vi "GapWeight.vi"(11 "GIC Input":T2={"     Use ?\nOff       On"=[FALSE, TRUE, FALSE, TRUE], "Mode:"=FALSE, "Extra Port"="", "Hokuyo Port"="COM7", "Tx Prop  Port"="COM6", "Compass Port"="", "GPS Port"="", "Num of WPs"=0, "WP Lats and Longs"={"WP Lats"=[], "WP Longs"=[]}, "Obst Lats and Longs"={"Obst Lats"=[], "Obst Longs"=[]}, "Parameters"=[], "GPS Data"=[], "Compass"=0.0, "LMS Vector"=[], "Vision Vector"=[], "Direction Cmd"=0.0, "Speed Cmd"=0.0, "WP Vector"=[], "WP Number"=0, "Extra"=0, "SW Map"=[], "Path Cluster"={"Path x node"=[], "Path y node"=[]}, "Sim Course"=[]} {"Obst Lats and Longs"."Obst Longs" format="%#_8g"; "Obst Lats and Longs"."Obst Lats" format="%#_8g"}) -> (3 "GIC Output":T1={"     Use ?\nOff       On"=[FALSE, TRUE, FALSE, TRUE], "Mode:"=FALSE, "Extra Port"="", "Hokuyo Port"="COM7", "Tx Prop Port"="COM6", "Compass Port"="", "GPS Port"="", "Num of WPs"=0, "WP Lats and Longs"={"WP Lats"=[], "WP Longs"=[]}, "Obst Lats and Longs"={"Obst Lats"=[], "Obst Longs"=[]}, "Parameters"=[], "GPS Data"=[], "Compass"=0.0, "LMS Vector"=[], "Vision Vector"=[], "Direction Cmd"=0.0, "Speed Cmd"=0.0, "WP Vector"=[], "WP Number"=0, "Extra"=0, "SW Map"=[], "Path Cluster"={"Path x node"=[], "Path y node"=[]}, "Sim Course"=[]} {"Obst Lats and Longs"."Obst Longs" format="%#_8g"; "Obst Lats and Longs"."Obst Lats" format="%#_8g"})   [LabVIEW 2014]
panel:
  out "nr":dbl
  out "nl":dbl
  out "Wr67":dbl
  out "Wl67":dbl
  out "lr67":dbl
  out "ll67":dbl
  out "sr67":dbl
  out "sl67":dbl
  out "tr67":dbl
  out "tl67":dbl
  out "dr67":dbl
  out "dl67":dbl
  out "Wr90":dbl
  out "Wr45":dbl
  out "Wr23":dbl
  out "W0":dbl
  out "Wl23":dbl
  out "Wl45":dbl
  out "Wl90":dbl
  out "lr90":dbl
  out "lr45":dbl
  out "lr23":dbl
  out "l0":dbl
  out "ll23":dbl
  out "ll45":dbl
  out "ll90":dbl
  out "sr90":dbl
  out "sr45":dbl
  out "sr23":dbl
  out "s0":dbl
  out "sl23":dbl
  out "sl45":dbl
  out "sl90":dbl
  out "tr90":dbl
  out "tr45":dbl
  out "tr23":dbl
  out "t0":dbl
  out "tl23":dbl
  out "tl45":dbl
  out "tl90":dbl
  out "Conf":dbl
  out "Slant":dbl
  out "drW":dbl
  out "dr45W":dbl
  out "dr23W":dbl
  out "d0W":dbl
  out "dl23W":dbl
  out "dl45W":dbl
  out "dlW":dbl
  out "wpvector":dbl[](array[numeric])
  out "ya":dbl
  out "xa":dbl
  out "dl23":dbl
  out "dr23":dbl
  out "a":dbl
  out "s":dbl
  out "objy":dbl
  out "objx":dbl
  out "dl":dbl
  out "dr":dbl
  out "dl45":dbl
  out "dr45":dbl
  out "d0":dbl
  # "GapWeight"
  # "Input:"
  # "Output"
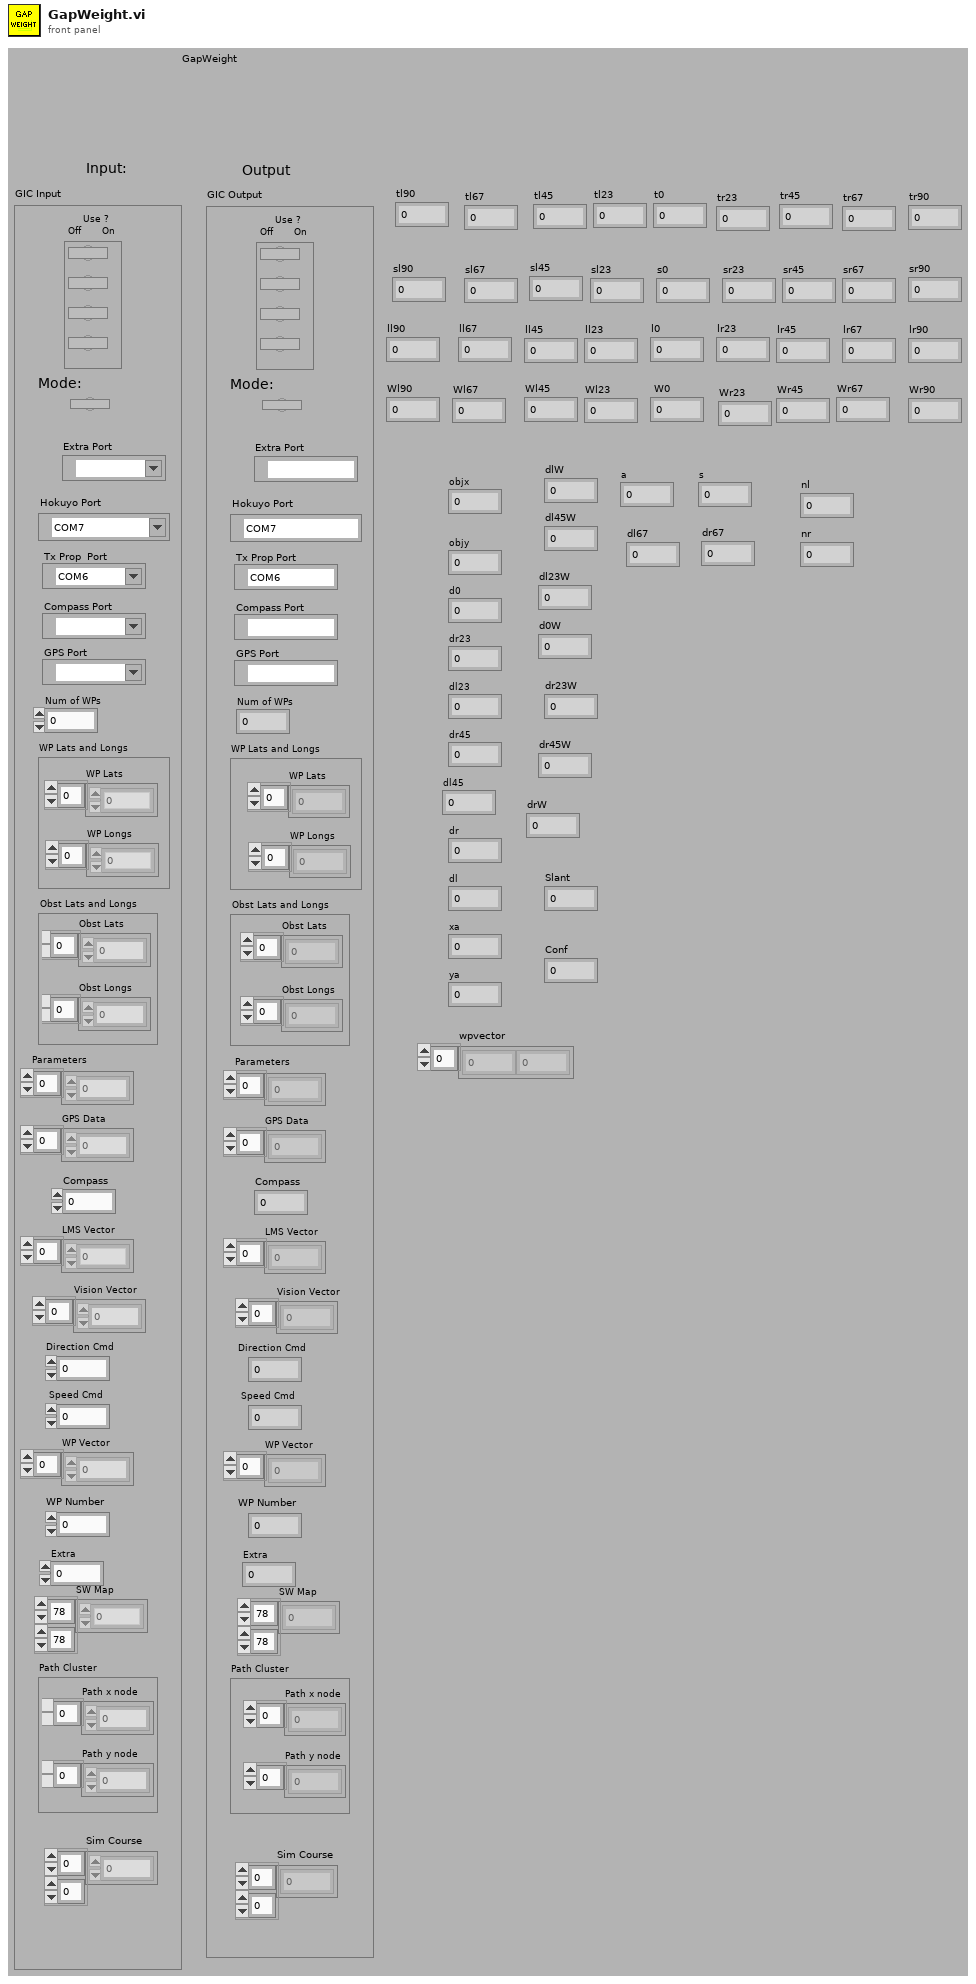
[diagram p1: front panel]
types:
  T1 = cluster{"     Use ?\nOff       On":bool[], "Mode:":bool, "Extra Port":refnum<visa-resource-name>, "Hokuyo Port":refnum<visa-resource-name>, "Tx Prop Port":refnum<visa-resource-name>, "Compass Port":refnum<visa-resource-name>, "GPS Port":refnum<visa-resource-name>, "Num of WPs":i16, "WP Lats and Longs":cluster{"WP Lats":dbl[], "WP Longs":dbl[]}, "Obst Lats and Longs":cluster{"Obst Lats":dbl[], "Obst Longs":dbl[]}, "Parameters":dbl[], "GPS Data":dbl[], "Compass":dbl, "LMS Vector":dbl[], "Vision Vector":dbl[], "Direction Cmd":dbl, "Speed Cmd":dbl, "WP Vector":dbl[], "WP Number":i32, "Extra":i16, "SW Map":i32[][], "Path Cluster":cluster{"Path x node":dbl[], "Path y node":dbl[]}, "Sim Course":i8[][]}
  T2 = cluster{"     Use ?\nOff       On":bool[], "Mode:":bool, "Extra Port":refnum<visa-resource-name>, "Hokuyo Port":refnum<visa-resource-name>, "Tx Prop  Port":refnum<visa-resource-name>, "Compass Port":refnum<visa-resource-name>, "GPS Port":refnum<visa-resource-name>, "Num of WPs":i16, "WP Lats and Longs":cluster{"WP Lats":dbl[], "WP Longs":dbl[]}, "Obst Lats and Longs":cluster{"Obst Lats":dbl[], "Obst Longs":dbl[]}, "Parameters":dbl[], "GPS Data":dbl[], "Compass":dbl, "LMS Vector":dbl[], "Vision Vector":dbl[], "Direction Cmd":dbl, "Speed Cmd":dbl, "WP Vector":dbl[], "WP Number":i32, "Extra":i16, "SW Map":i32[][], "Path Cluster":cluster{"Path x node":dbl[], "Path y node":dbl[]}, "Sim Course":i8[][]}
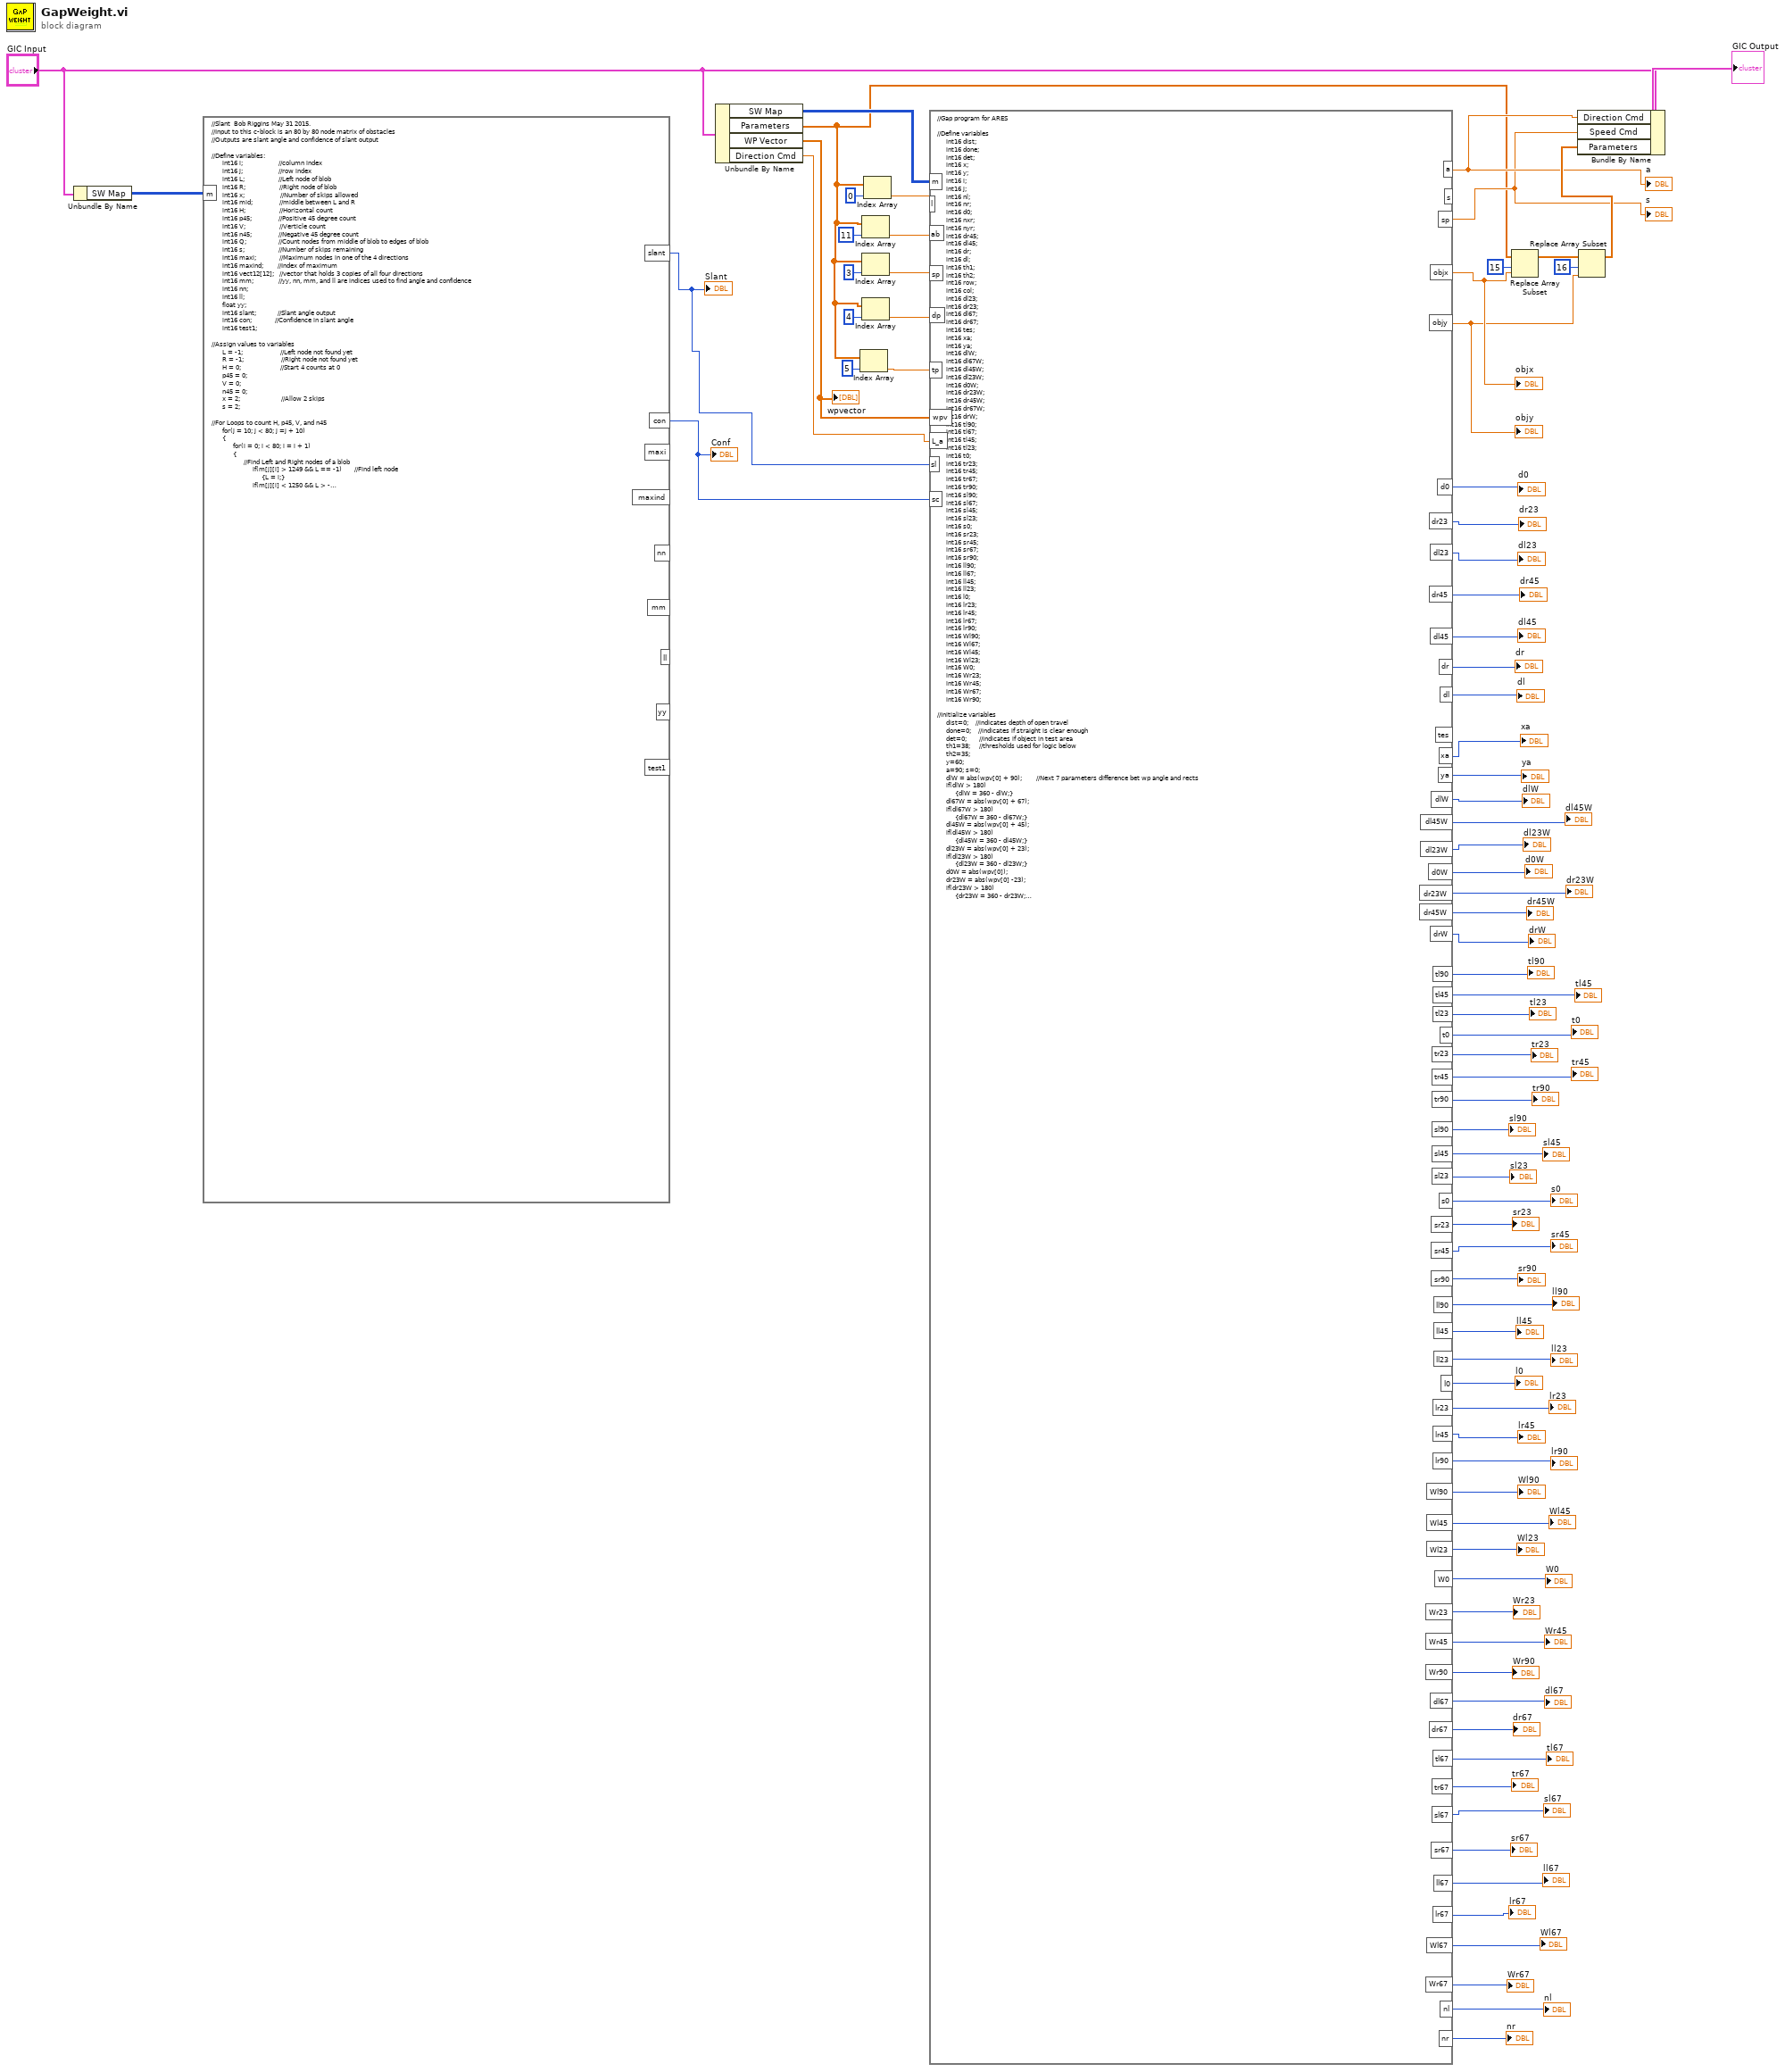
[diagram p0: block diagram]
diagram:
  n1 = Unbundle By Name("GIC Input") -> ("SW Map"=w52:i32[][])
  n2 = formula code="//Slant  Bob Riggins May 31 2015.  \n//Input to this c-block is an 80 by 80 node matrix of obstacles\n//Outputs are slant angle and confidence of slant output\n\n//Define variables:\n      int16 i;                    //column index\n      int16 j;                    //row index\n      int16 L;                   //Left node of blob\n      int16 R;                   //Right node of blob\n      int16 x;                    //Number of skips allowed\n      int16 mid;               //middle between L and R\n      int16 H;                   //Horizontal count\n      int16 p45;               //Positive 45 degree count\n      int16 V;                   //Verticle count\n      int16 n45;               //Negative 45 degree count\n      int16 Q;                  //Count nodes from middle of blob to edges of blob\n      int16 s;                   //Number of skips remaining\n      int16 maxi;             //Maximum nodes in one of the 4 directions\n      int16 maxind;        //Index of maximum\n      int16 vect12[12];   //vector that holds 3 copies of all four directions\n      int16 mm;              //yy, nn, mm, and ll are indices used to find angle and confidence\n      int16 nn;\n      int16 ll;\n      float yy;\n      int16 slant;            //Slant angle output\n      int16 con;             //Confidence in slant angle\n      int16 test1;\n\n//Assign values to variables\n      L = -1;                     //Left node not found yet\n      R = -1;                     //Right node not found yet\n      H = 0;                      //Start 4 counts at 0\n      p45 = 0;\n      V = 0;\n      n45 = 0;\n      x = 2;                       //Allow 2 skips\n      s = 2;\n\n//For Loops to count H, p45, V, and n45\n      for(j = 10; j < 80; j =j + 10)\n      {\n            for(i = 0; i < 80; i = i + 1)\n            {\n                  //Find Left and Right nodes of a blob\n                       if(m[j][i] > 1249 && L == -1)       //Find left node\n                            {L = i;}\n                       if(m[j][i] < 1250 && L > -1 && s == 0)          //Find right node\n                            {R = i - 1 - x;} \n                       if(m[j][i] <1250 && L > -1 && s > 0)         //Allow for skips\n                            {s = s - 1;}\n                       if(i == 79 && m[j][i] > 1249 && L == -1)      //single node at edge\n                       {                                                                            //define L and R there\n                             L == 79;\n                             R == 79;\n                       }       \n                       if(i == 79 && m[j][i] > 1249 && L > -1)       //blob at edge (L found)\n                            {R = 79;}   \n                       if(i == 79 && m[j][i] < 1250 && L > -1)       //blob at edge (L found)\n                            {R = 78;}\n\n                       if(L > -1 && R > -1)         //If L and R exist then start counting from mid\n                       {\n                            H = H + (R - L);                         //Updated H\n                            if(j==10)\n                                 {test1 = R;}\n                            mid = int((L + R)/2);                //Set up middle of blob for counting\n                            L = -1;\n                            R = -1;\n                            s = x;\n                            Q = 1; \n                \n                       //Count N45 (negative 45 degrees thru mid of blob)\n                            while (s > 0 && j + Q < 80 && mid + Q < 80)\n                                {\n                                     while (m[j + Q][mid + Q] > 1249)    //Count down and to right\n                                          {\n                                               n45 = n45 + 1;\n                                               s = x;\n                                               Q = Q + 1;\n                                          }\n                                     while (m[j + Q][mid + Q] < 1250 && s > 0)   //Allow x skips\n                                          {\n                                               n45 = n45 + 1;\n                                               s = s - 1;\n                                               Q = Q + 1;\n                                          }\n                                }     //end of while loop for counting n45 down and to right\n                                n45 = n45 - x;\n                                s = x;\n                                Q = 1;\n\n                                while (s > 0 && j - Q > -1 && mid - Q > -1)\n                                {\n                                     while (m[j - Q][mid - Q] > 1249)    //Count up and to left\n                                          {\n                                               n45 = n45 + 1;\n                                               s = x;\n                                               Q = Q + 1;\n                                          }\n                                     while (m[j - Q][mid - Q] < 1250 && s > 0)   //Allow x skips\n                                          {\n                                               n45 = n45 + 1;\n                                               s = s - 1;\n                                               Q = Q + 1;\n                                          }\n                                }     //end of while loop for counting n45 up and to left\n                                n45 = n45 - x;\n                                s = x;\n                                Q = 1;\n\n                       //Count V (verticle thru mid of blob)\n                            while (s > 0 && j + Q < 80)\n                                {\n                                     while (m[j + Q][mid] > 1249)    //Count down from mid\n                                          {\n                                               V = V + 1;\n                                               s = x;\n                                               Q = Q + 1;\n                                          }\n                                     while (m[j + Q][mid] < 1250 && s > 0)   //Allow x skips\n                                          {\n                                               V = V + 1;\n                                               s = s - 1;\n                                               Q = Q + 1;\n                                          }\n                                }     //end of while loop for counting V down\n                                V = V - x;\n                                s = x;\n                                Q = 1;\n\n                                while (s > 0 && j - Q > -1)\n                                {\n                                     while (m[j - Q][mid] > 1249)    //Count up\n                                          {\n                                               V = V + 1;\n                                               s = x;\n                                               Q = Q + 1;\n                                          }\n                                     while (m[j - Q][mid] < 1250 && s > 0)   //Allow x skips\n                                          {\n                                               V = V + 1;\n                                               s = s - 1;\n                                               Q = Q + 1;\n                                          }\n                                }     //end of while loop for counting V up\n                                V = V - x;\n                                s = x;\n                                Q = 1;\n\n                       //Count p45 (positive 45 degrees thru mid of blob)\n                            while (s > 0 && j + Q < 80 && mid - Q > -1)\n                                {\n                                     while (m[j + Q][mid - Q] > 1249)    //Count down and to left\n                                          {\n                                               p45 = p45 + 1;\n                                               s = x;\n                                               Q = Q + 1;\n                                          }\n                                     while (m[j + Q][mid - Q] < 1250 && s > 0)   //Allow x skips\n                                          {\n                                               p45 = p45 + 1;\n                                               s = s - 1;\n                                               Q = Q + 1;\n                                          }\n                                }     //end of while loop for counting p45 down and to left\n                                p45 = p45 - x;\n                                s = x;\n                                Q = 1;\n\n                                while (s > 0 && j - Q > -1 && mid + Q < 80)\n                                {\n                                     while (m[j - Q][mid + Q] > 1249)    //Count up and to right\n                                          {\n                                               p45 = p45 + 1;\n                                               s = x;\n                                               Q = Q + 1;\n                                          }\n                                     while (m[j - Q][mid + Q] < 1250 && s > 0)   //Allow x skips\n                                          {\n                                               p45 = p45 + 1;\n                                               s = s - 1;\n                                               Q = Q + 1;\n                                          }\n                                }     //end of while loop for counting p45 up and to right\n                                p45 = p45 - x;\n                                s = x;\n                                Q = 1;\n\n                       }                                                    //end of IF for counts for blob\n            }                                    //end of FOR for i\n      }                                          //end of FOR for j\n      \n      //Now have H, p45, V, n45.  Find slan and con  (slant angle and confidence)\n            maxi = H;                                   //Initialize process of finding maximum direction\n            maxind = 0;\n            if(p45 > maxi)\n            {\n                 maxi = p45;\n                 maxind = 1;\n            }\n            if(V > maxi)\n            {\n                 maxi = V;\n                 maxind = 2;\n            }\n            if(n45 > maxi)\n            {\n                 maxi = n45;\n                 maxind = 3;\n            }                                                    //now, max value of 4 directions in maxi\n                                                                 //maxind is index of direction of max\n\n            for(i = 0; i < 3; i = i + 1)            //Next, make vect12, 3 copies of 4 directions\n            {\n                 vect12[4*i] = H;\n                 vect12[4*i + 1] = p45;\n                 vect12[4*i + 2] = V;\n                 vect12[4*i + 3] = n45;\n            }\n           \n            if(maxi != 0)\n            {\n                 nn = vect12[maxind - 1];                          //Use max direction and \"pull\" off to sides\n                 mm = vect12[maxind + 1];\n                 ll = vect12[maxind + 2];\n                 yy = (mm - nn)/(maxi + mm + mm);\n                 con = (1 - (ll/maxi)) * 100;                                    //Confidence of slant calculation\n\n                 if(maxind == 0)                                         //Find slant angle\n                    {slant = 45 * yy;}\n                 if(maxind == 1)                                         \n                    {slant = 45 * (1 - yy);}\n                 if(maxind == 2)                                         \n                    {slant = (45 * (1 - yy)) - 45;}\n                 if(maxind == 3)                                         \n                    {slant = -45 * (1 + yy);}\n             }\n\n             if(maxi == 0)\n             {\n                  slant = 0;\n                  con = 0;\n             }"("m"=w52) -> ("slant"=w51:i16, "con"=w50:i16)  [unwired: 7 out]
  "Slant" <- w51
  "Conf" <- w50
  n3 = Unbundle By Name("GIC Input") -> ("SW Map"=w83:i32[][], "Parameters"=w44:dbl[], "WP Vector"=w49:dbl[], "Direction Cmd"=w1:dbl)
  "wpvector" <- w49
  n4 = Index Array(array=w44, index=5) -> (element=w42:dbl)
  n5 = Index Array(array=w44, index=11) -> (element=w63:dbl)
  n6 = Index Array(array=w44, index=3) -> (element=w47:dbl)
  n7 = Index Array(array=w44, index=4) -> (element=w45:dbl)
  n8 = Index Array(array=w44, index=0) -> (element=w81:dbl)
  n9 = formula code="//Gap program for ARES\n\n//Define variables\n     int16 dist;\n     int16 done;\n     int16 det;\n     int16 x;\n     int16 y;\n     int16 i;\n     int16 j;\n     int16 nl;\n     int16 nr;\n     int16 d0;\n     int16 nxr;\n     int16 nyr;\n     int16 dr45;\n     int16 dl45;\n     int16 dr;\n     int16 dl;\n     int16 th1;\n     int16 th2;\n     int16 row;\n     int16 col;\n     int16 dl23;\n     int16 dr23;\n     int16 dl67;\n     int16 dr67;\n     int16 tes;\n     int16 xa;\n     int16 ya;\n     int16 dlW;\n     int16 dl67W;\n     int16 dl45W;\n     int16 dl23W;\n     int16 d0W;\n     int16 dr23W;\n     int16 dr45W;\n     int16 dr67W;\n     int16 drW;\n     int16 tl90;\n     int16 tl67;\n     int16 tl45;\n     int16 tl23;\n     int16 t0;\n     int16 tr23;\n     int16 tr45;\n     int16 tr67;\n     int16 tr90;\n     int16 sl90;\n     int16 sl67;\n     int16 sl45;\n     int16 sl23;\n     int16 s0;\n     int16 sr23;\n     int16 sr45;\n     int16 sr67;\n     int16 sr90;\n     int16 ll90;\n     int16 ll67;\n     int16 ll45;\n     int16 ll23;\n     int16 l0;\n     int16 lr23;\n     int16 lr45;\n     int16 lr67;\n     int16 lr90;\n     int16 Wl90;\n     int16 Wl67;\n     int16 Wl45;\n     int16 Wl23;\n     int16 W0;\n     int16 Wr23;\n     int16 Wr45;\n     int16 Wr67;\n     int16 Wr90;\n\n//Initialize variables\n     dist=0;    //indicates depth of open travel\n     done=0;    //indicates if straight is clear enough\n     det=0;       //indicates if object in test area\n     th1=38;     //thresholds used for logic below\n     th2=35;\n     y=60;\n     a=90; s=0;\n     dlW = abs(wpv[0] + 90);        //Next 7 parameters difference bet wp angle and rects\n     if(dlW > 180)\n          {dlW = 360 - dlW;}\n     dl67W = abs(wpv[0] + 67);\n     if(dl67W > 180)\n          {dl67W = 360 - dl67W;}\n     dl45W = abs(wpv[0] + 45);\n     if(dl45W > 180)\n          {dl45W = 360 - dl45W;}\n     dl23W = abs(wpv[0] + 23);\n     if(dl23W > 180)\n          {dl23W = 360 - dl23W;}\n     d0W = abs(wpv[0]);\n     dr23W = abs(wpv[0] -23);\n     if(dr23W > 180)\n          {dr23W = 360 - dr23W;}\n     dr45W = abs(wpv[0] -45);\n     if(dr45W > 180)\n          {dr45W = 360 - dr45W;}\n     dr67W = abs(wpv[0] -67);\n     if(dr67W > 180)\n          {dr67W = 360 - dr67W;}\n     drW = abs(wpv[0] - 90);\n     if(drW > 180)\n          {drW = 360 - drW;}\n\n//Count obstacles to immediate left and right for weight info\n//Number of objects on left is nl and on right nr.\n     nl = 0; nr = 0;\n     for(i = 1; i< 10; i = i + 1)\n     {\n          for(j = 1; j< 10; j = j + 1)\n          {\n               if(m[60 - j][40 - i] > 1249)\n               {nl = nl + 1;}\n               if(m[60 - j][40 + i] > 1249)  \n               {nr = nr + 1;}\n          }\n     }   \n\n//Test rectangle in front. Check for obstacles\n     while(det==0 && y>=1)\n     {\n          y=60-dist;\n          x=40-l;\n          while (x<= 40+l && det==0)\n          {\n               if (m[y][x]>=2500)\n                    {det=1;}\n               x=x+1;\n          }\n          dist=dist+1;\n     }\n     d0=dist-1;     //d0 is how far it can move forward\n\n//Test rectangle at 23 degrees to left\n     //Set variables\n          dist=0;det=0;nxr=40;row=0;x=40;y=60;\n     //Check for obstacles\n          while(det==0 && x>2+2*l && y>=1)\n          {\n               x=nxr-l;\n               if(row==0)\n               {\n                    while(x<=nxr+l && det==0)\n                    {\n                         if((y!=60 && y!=59) || x!=40+l)\n                         {\n                              if(m[y][x]>=2500)\n                                   {det=1;}\n                         }\n                         x=x+1;\n                    }\n                    row=1;dist=dist+1;y=y-1;\n               }\n               else\n               {\n                     while(x<=nxr+l && det==0)\n                    {\n                         if((y!=60 && y!=59) || x!=40+l)\n                         {\n                              if(m[y][x]>=2500)\n                                   {det=1;}\n                         } \n                         x=x+1;\n                   }\n                    row=0;dist=dist+1;y=y-1; nxr=nxr-1;\n              }  \n          }  \n          dl23=dist-1;  \n\n//Test rectangle at 23 degrees to right\n     //Set variables\n          dist=0;det=0;nxr=40;row=0;x=40;y=60;\n     //Check for obstacles\n          while(det==0 && x<=77 && y>=1)\n          {\n               x=nxr-l;\n               if(row==0)\n               {\n                    while(x<=nxr+l && det==0)\n                    {\n                         if((y!=60 && y!=59) || x!=40-l)\n                         {\n                              if(m[y][x]>=2500)\n                                   {det=1;}\n                         }\n                         x=x+1;\n                    }\n                    row=1;dist=dist+1;y=y-1;\n               }\n               else\n               {\n                      while(x<=nxr+l && det==0)\n                    {\n                         if((y!=60 && y!=59) || x!=40-l)\n                         {\n                              if(m[y][x]>=2500)\n                                   {det=1;}\n                         }\n                         x=x+1;\n                    }\n                    row=0;dist=dist+1;y=y-1; nxr=nxr+1;\n               }\n          }\n          dr23=dist-1;   \n\n//Test rectangle at 67 degrees to right\n     //Set variables\n          dist=0;det=0;nyr=60;col=0;x=40;y=60;\n     //Check for obstacles\n          while(det==0 && x< 80-l)\n          {\n               y=nyr-l;\n               if(col==0)\n               {\n                    while(y<=nyr+l && det==0)\n                    {\n                         if((x!=40 && x!=39) || y!=60+l)\n                         {\n                              if(m[y][x]>=2500)\n                                   {det=1;}\n                         }\n                         y=y+1;\n                    }\n                    col=1;dist=dist+1;x=x+1;\n               }\n               else\n               {\n                      while(y<=nyr+l && det==0)\n                    {\n                         if((x!=40 && x!=39) || y!=60+l)\n                         {\n                              if(m[y][x]>=2500)\n                                   {det=1;}\n                         }\n                         y=y+1;\n                    }\n                    col=0;dist=dist+1;x=x+1; nyr=nyr-1;\n               }\n          }\n          dr67=(dist-1) * 1.086;   \n\n//If room to the front or 23 degree to either side, just go there\n     //if(d0>=th1 || dr23>=th1 || dl23>=th1)\n          //{done=1;}\n\n//Test rectangle at 45 degrees to right\n     //Set variables\n          dist=0;det=0;nxr=40;nyr=60;x=40;\n     //Check for obstacles\n          while(det==0 && x<=77)\n          {\n               x=nxr-l; y=nyr-l;\n               while(x<=nxr+l && det==0)\n                    {\n                         if(m[y][x]>=2500)\n                              {det=1;}\n                         if(m[y-1][x]>=2500)\n                              {det=1;}\n                         if(x==nxr+l)\n                         {\n                              if(m[y][x+1]>=2500)\n                                   {det=1;}\n                         }\n                         x=x+1; y=y+1;\n                    }\n                    nxr=nxr+1;nyr=nyr-1;\n                    dist=dist+1;\n          }\n          dr45=(dist-1)*1.616;\n\n//Test rectangle at 45 degrees to left\n     //Set variables\n          dist=0;det=0;nxr=40;nyr=60;x=40;\n     //Check for obstacles\n          while(det==0 && x>=2+2*l)\n          {\n               x=nxr-l; y=nyr+l;\n               while(x<=nxr+l && det==0)\n                    {\n                         if(m[y][x]>=2500)\n                              {det=1;}\n                         if(m[y][x-1]>=2500)\n                              {det=1;}\n                         if(x==nxr+l)\n                         {\n                              if(m[y-1][x]>=2500)\n                                   {det=1;}\n                         }\n                         x=x+1; y=y-1;\n                    }\n                    nxr=nxr-1;nyr=nyr-1;\n                    dist=dist+1;\n          }\n          dl45=(dist-1)*1.4886;   \n\n//Test rectangle at 67 degrees to left\n     //Set variables\n          dist=0;det=0;nyr=60;col=0;x=40;y=60;\n     //Check for obstacles\n          while(det==0 && x>l)\n          {\n               y=nyr-l;\n               if(col==0)\n               {\n                    while(y<=nyr+l && det==0)\n                    {\n                         if((x!=40 && x!=39) || y!=60+l)\n                         {\n                              if(m[y][x]>=2500)\n                                   {det=1;}\n                         }\n                         y=y+1;\n                    }\n                    col=1;dist=dist+1;x=x-1;\n               }\n               else\n               {\n                     while(y<=nyr+l && det==0)\n                    {\n                         if((x!=40 && x!=39) || y!=60+l)\n                         {\n                              if(m[y][x]>=2500)\n                                   {det=1;}\n                         } \n                         y=y+1;\n                   }\n                    col=0;dist=dist+1;x=x-1; nyr=nyr-1;\n              }  \n          }  \n          dl67=(dist-1) * 1.086;  \n\n//Test rectangle to the right (right below and above robot)\n     //Set variables\n          dist=0;det=0; x=0;\n          while(det==0 && x<=78)\n          {\n               x=40+dist; y=60+l;\n               while(y>=60-l && det==0)\n               {\n                    if (m[y][x] >=2500)\n                         {det=1;}\n                    y=y-1;\n               }\n               dist=dist+1;\n          }\n          dr=(dist-1)*1.0256;\n\n//Test rectangle to the left (left below and above robot)\n     //Set variables\n          dist=0;det=0; x=1;\n          while(det==0 && x>=1)\n          {\n               x=40-dist; y=60+l;\n               while(y>=60-l && det==0)\n               {\n                    if (m[y][x] >=2500)\n                         {det=1;}\n                    y=y-1;\n               }\n               dist=dist+1;\n          }\n          dl=dist-1;\n\n//If WP dist is less than a rectangle dist that is closest in angle to wp, go that way\n//Else if rect angle that is closest to wp has dist at least th1, go that way\n     if (dlW < dl67W && dlW < dl45W && dlW < dl23W && dlW < d0W && dlW < dr23W && dlW < dr45W && dlW < dr67W && dlW < drW)\n          {\n               if ( dl >= wpv[1] * 10)\n                    {s = dl; a = 90 - wpv[0]; done = 1;}\n          } \n     if (dl67W < dlW && dl67W < dl45W && dl67W < dl23W && dl67W < d0W && dl67W < dr23W && dl67W < dr45W && dl67W < dr67W && dl67W < drW)\n          {\n               if ( dl45 >= wpv[1] * 10)\n                    {s = dl67; a = 90 - wpv[0]; done = 1;}\n          }   \n     if (dl45W < dlW && dl45W < dl67W && dl45W < dl23W && dl45W < d0W && dl45W < dr23W && dl45W < dr45W && dl45W < dr67W && dl45W < drW)\n          {\n               if ( dl45 >= wpv[1] * 10)\n                    {s = dl45; a = 90 - wpv[0]; done = 1;}\n          }   \n     if (dl23W < dlW && dl23W < dl67W && dl23W < dl45W && dl23W < d0W && dl23W < dr23W && dl23W < dr45W && dl23W < dr67W && dl23W < drW)\n          {\n               if ( dl23 >= wpv[1] * 10)\n                    {s = dl23; a = 90 - wpv[0]; done = 1;}\n          } \n     if (d0W < dlW && d0W < dl67W && d0W < dl45W && d0W < dl23W && d0W < dr23W && d0W < dr45W && d0W < dr67W && d0W < drW)\n          {\n               if ( d0 >= wpv[1] * 10)\n                    {s = d0; a = 90 - wpv[0]; done = 1;}\n          } \n     if (dr23W < dlW && dr23W < dl67W && dr23W < dl45W && dr23W < dl23W && dr23W < d0W && dr23W < dr45W && dr23W < dr67W && dr23W < drW)\n          {\n               if ( dr23 >= wpv[1] *  10)\n                    {s = dr23; a = 90 - wpv[0]; done = 1;}\n          } \n     if (dr45W < dlW && dr45W < dl67W && dr45W < dl45W && dr45W < dl23W && dr45W < d0W && dr45W < dr23W && dr45W < dr67W && dr45W < drW)\n          {\n               if ( dr45>= wpv[1] * 10)\n                    {s = dr45; a = 90 - wpv[0]; done = 1;}\n          } \n     if (dr67W < dlW && dr67W < dl67W && dr67W < dl45W && dr67W < dl23W && dr67W < d0W && dr67W < dr23W && dr67W < dr45W && dr67W < drW)\n          {\n               if ( dr45>= wpv[1] * 10)\n                    {s = dr67; a = 90 - wpv[0]; done = 1;}\n          } \n     if (drW < dlW && drW < dl67W && drW < dl45W && drW < dl23W && drW < d0W && drW < dr23W && drW < dr45W && drW < dr67W)\n          {\n               if ( dr>= wpv[1] * 10)\n                    {s = dr; a = 90 - wpv[0]; done = 1;}\n          } \n     if (done ==1)\n          {\n               objx=40+cos(a*0.017453)*s;\n               objy=60-sin(a*0.017453)*s;\n          }\n\n//If no direct path to wp on local map then weight the gaps\n     if(done == 0)\n          {\n               if(nl + nr > 20)\n                    {tp = 0; sp = 0;}\n\n               tl90 = (100 - (dlW*100)/180) * tp;\n               tl67 = (100 - (dl67W*100)/180) * tp;\n               tl45 = (100 - (dl45W*100)/180) * tp;\n               tl23 = (100 - (dl23W*100)/180) * tp;\n               t0 = (100 - (d0W*100)/180) * tp;\n               tr23 = (100 - (dr23W*100)/180) * tp;\n               tr45 = (100 - (dr45W*100)/180) * tp;\n               tr67 = (100 - (dr67W*100)/180) * tp;\n               tr90 = (100 - (drW*100)/180) * tp;\n               \n               if(sc<60)\n                    {sp = 0;;}\n\n               sl90 = ((1 - sin(sl*3.14159/180))*(sc/2)) * sp;\n               sl67= ((-.9205*sin(sl*3.14159/180) + .39073 * cos(sl*3.14159/180) + 1) * (sc/2)) * sp;\n               sl45= ((-.707*sin(sl*3.14159/180) + .707 * cos(sl*3.14159/180) + 1) * (sc/2)) * sp;\n               sl23= ((-.39073*sin(sl*3.14159/180) + .9205 * cos(sl*3.14159/180) + 1) * (sc/2)) * sp;\n               s0 = ((cos(sl*3.14159/180) + 1) * (sc/2)) * sp;\n               sr23= ((.39073*sin(sl*3.14159/180) + .9205 * cos(sl*3.14159/180) + 1) * (sc/2)) * sp;\n               sr45= ((.707*sin(sl*3.14159/180) + .707 * cos(sl*3.14159/180) + 1) * (sc/2)) * sp;\n               sr67= ((.9205*sin(sl*3.14159/180) + .39073 * cos(sl*3.14159/180) + 1) * (sc/2)) * sp;\n               sr90 = ((1 + sin(sl*3.14159/180))*(sc/2)) * sp;\n\n               //ll90 = ((dl * 100)/40) * dp;\n               //ll67 = ((dl67 * 100)/40) * dp;\n               //ll45 = ((dl45 * 100)/57) * dp;\n               //ll23 = ((dl23 * 100)/59) * dp;\n               //l0 = ((d0 * 100)/60) * dp;\n               //lr23 = ((dr23 * 100)/59) * dp;\n               //lr45 = ((dr45 * 100)/57) * dp;\n               //lr67 = ((dr67 * 100)/40) * dp;\n               //lr90 = ((dr * 100)/40) * dp;\n\n               ll90 = (dl * 100)/60 * dp;\n               ll67 = (dl67 * 100)/60 * dp;\n               ll45 = ((dl45 * 100)/60) * dp;\n               ll23 = ((dl23 * 100)/60) * dp;\n               l0 = ((d0 * 100)/60) * dp;\n               lr23 = ((dr23 * 100)/60) * dp;\n               lr45 = ((dr45 * 100)/60) * dp;\n               lr67 = ((dr67 * 100)/60) * dp;\n               lr90 = ((dr * 100)/60) * dp;\n\n               Wl90 = tl90 + sl90 + ll90;\n               Wl67 = tl67 + sl67 + ll67;\n               Wl45 = tl45 + sl45 + ll45;\n               Wl23 = tl23 + sl23 + ll23;\n               W0 = t0 + s0 + l0;\n               Wr23 = tr23 + sr23 + lr23;\n               Wr45 = tr45 + sr45 + lr45;\n               Wr67 = tr67 + sr67 + lr67;\n               Wr90 = tr90 + sr90 + lr90;\n\n          }\n\n           \n//Go in direction of biggest weight at speed proportional to distance\n     if(done == 0)\n          {\n          if(d0>th2 || dr67 > th2 || dr45 >th2 || dl45>th2 || dl67 > th2 || dr>th2 || dl>th2 || dr23>th2 || dl23>th2)\n          {\n               if(Wl90 >= Wl67 && Wl90>=Wl45 && Wl90>=Wl23 && Wl90>= W0 && Wl90>=Wr23 && Wl90>=Wr45 && Wl90>=Wr67 && Wl90>= Wr90)\n                    {s=dl;a=180;}\n               if(Wl67 >= Wl90 && Wl67>=Wl45 && Wl67>=Wl23 && Wl67 >= W0 && Wl67 >=Wr23 && Wl67 >=Wr45 && Wl67 >=Wr67 && Wl67 >= Wr90)\n                    {s=dl67;a=157 + (dl - dl45)/3;}\n               if(Wl45>=Wl90 && Wl45 >= Wl67 && Wl45>=Wl23 && Wl45>= W0 && Wl45>=Wr23 && Wl45>=Wr45 && Wl45>=Wr67 && Wl45>= Wr90)\n                    {s=dl45;a=135 + (dl67 - dl23)/3;}\n               if(Wl23>=Wl90 && Wl23>=Wl67 && Wl23>=Wl45 && Wl23>= W0 && Wl23>=Wr23 && Wl23>=Wr45 && Wl23>=Wr67 &&Wl23>= Wr90)\n                    {s=dl23;a=113 + (dl45 - d0)/3;}\n               if(W0>=Wl90 && W0>=Wl67 && W0>=Wl45 && W0>= Wl23 && W0>=Wr23 && W0>=Wr45 && W0>=Wr67 && W0>= Wr90)\n                    {s=d0;a=90 + (dl23 - dr23)/3;}\n               if(Wr23>=Wl90 && Wr23>=Wl67 && Wr23>=Wl45 && Wr23>= Wl23 && Wr23>=W0 && Wr23>=Wr45 && Wr23>=Wr67 && Wr23>= Wr90)\n                    {s=dr23;a=67 + (d0 - dr45)/3;}\n               if(Wr45>=Wl90 && Wr45>=Wl67 && Wr45>=Wl45 && Wr45>= Wl23 && Wr45>=W0 && Wr45>=Wr23 && Wr45>=Wr67 && Wr45>= Wr90)\n                    {s=dr45;a=45 + (dr23 - dr67)/3;}\n               if(Wr67>=Wl90 && Wr67>=Wl67 && Wr67>=Wl45 && Wr67>= Wl23 && Wr67>=W0 && Wr67>=Wr23 && Wr67>=Wr45 && Wr67>= Wr90)\n                    {s=dr67;a= 23 + (dr45 - dr)/3;}\n               if(Wr90>=Wl90 && Wr90>=Wl67 && Wr90>=Wl45 && Wr90>= Wl23 && Wr90>=W0 && Wr90>=Wr23 && Wr90>= Wr45 && Wr90>= Wr67)\n                    {s=dr;a=0;}\n\n\n//               if(d0>=dr45 && d0>=dl45 && d0>=dr && d0>=dl && d0>=dr23 && d0>= dl23)\n//                    {s=d0;a=90 + (dl23 - dr23)/3;}\n//               if(dr45>d0 && dr45>=dl45 && dr45>=dr && dr45>=dl && dr45>dr23 && dr45>dl23)\n//                    {s=dr45;a=45;}\n//               if(dl45>d0 && dl45>dr45 && dl45 >=dr && dl45>=dl && dl45>dr23 && dl45>dl23)\n//                    {s=dl45;a=135;}\n//               if(dr>d0 && dr>dr45 && dr>dl45 && dr>=dl && dr>dr23 && dr>dl23)\n//                    {s=dr;a=0;}\n//                if(dl>d0 && dl>dr45 && dl>dl45 && dl>dr && dl>dr23 && dl>dl23)\n//                    {s=dl;a=180;}\n//                if(dr23>d0 && dr23>=dl23 && dr23>=dr45 && dr23>=dl45 && dr23>=dr && dr23>=dl)\n//                    {s=dr23;a=67 + (d0 - dr45)/3;}\n//                if(dl23>d0 && dl23>dr23 && dl23>=dr45 && dl23>=dl45 && dl23>=dr && dl23>=dl)\n//                    {s=dl23;a=113 + (dl45 - d0)/3;}\n  \n                 if((L_a == 180)&&(a == 0))\n                      {a = 270; s = 10;}\n                 if((L_a == 0)&&(a == 180))\n                      {a = 270; s = 10;}\n                 //if((L_a - a) > 90)\n                 //      {a = 270; s = 10;}\n                 //if((a - L_a) > 90)\n                 //      {a = 270; s = 10;}\n\n                 objx=40+cos(a*0.017453)*s;\n                 objy=60-sin(a*0.017453)*s;\n          }\n          else\n               {\n                    s=30;a=270; objx=40; objy = 79;\n               }\n          }\n//Angle bias\n     a=a+ab;\n\n//Make speed command only the verticle component for sabertooth mixed mode\n     sp = (71* abs(objy - 60))/60;"("m"=w83, "l"=w81, "ab"=w63, "wpv"=w49, "sl"=w51, "sc"=w50, "sp"=w47, "dp"=w45, "tp"=w42, "L_a"=w1) -> ("a"=w69:dbl, "objx"=w71:dbl, "objy"=w70:dbl, "d0"=→"d0":i16, "dr45"=→"dr45":i16, "dl45"=→"dl45":i16, "dr"=→"dr":i16, "dl"=→"dl":i16, "dr23"=→"dr23":i16, "dl23"=→"dl23":i16, "xa"=→"xa":i16, "ya"=→"ya":i16, "sp"=w61:dbl, "dlW"=→"dlW":i16, "dl45W"=→"dl45W":i16, "dl23W"=→"dl23W":i16, "d0W"=→"d0W":i16, "dr23W"=→"dr23W":i16, "dr45W"=→"dr45W":i16, "drW"=→"drW":i16, "tl90"=→"tl90":i16, "tl45"=→"tl45":i16, "tl23"=→"tl23":i16, "t0"=→"t0":i16, "tr23"=→"tr23":i16, "tr45"=→"tr45":i16, "tr90"=→"tr90":i16, "sl90"=→"sl90":i16, "sl45"=→"sl45":i16, "sl23"=→"sl23":i16, "s0"=→"s0":i16, "sr23"=→"sr23":i16, "sr45"=→"sr45":i16, "sr90"=→"sr90":i16, "ll90"=→"ll90":i16, "ll45"=→"ll45":i16, "ll23"=→"ll23":i16, "l0"=→"l0":i16, "lr23"=→"lr23":i16, "lr45"=→"lr45":i16, "lr90"=→"lr90":i16, "Wl90"=→"Wl90":i16, "Wl45"=→"Wl45":i16, "Wl23"=→"Wl23":i16, "W0"=→"W0":i16, "Wr23"=→"Wr23":i16, "Wr45"=→"Wr45":i16, "Wr90"=→"Wr90":i16, "dl67"=→"dl67":i16, "dr67"=→"dr67":i16, "tl67"=→"tl67":i16, "tr67"=→"tr67":i16, "sl67"=→"sl67":i16, "sr67"=→"sr67":i16, "ll67"=→"ll67":i16, "lr67"=→"lr67":i16, "Wl67"=→"Wl67":i16, "Wr67"=→"Wr67":i16, "nl"=→"nl":i16, "nr"=→"nr":i16)  [unwired: 2 out]
  "objx" <- w71
  "objy" <- w70
  "s" <- w61
  "a" <- w69
  n10 = Replace Array Subset(array=w44, new element=w71, index=15) -> (w79:dbl[])
  n11 = Replace Array Subset(array=w79, new element=w70, index=16) -> (w77:dbl[])
  n12 = Bundle By Name(cluster="GIC Input", "Direction Cmd"=w69, "Speed Cmd"=w61, "Parameters"=w77) -> (→"GIC Output":T2)
